vi "I2C.vi"() -> ()   [LabVIEW 2017]
doc: "Utilisez ce modèle pour construire un modèle de conception producteur/consommateur avec des événements et des files d'attente. Ce modèle est préférable à celui du Gestionnaire d'événements de l'interface utilisateur parce qu'il permet au code de s'exécuter de façon asynchrone en réponse à un événement, sans ralentir le temps de réponse de l'interface utilisateur."
uses:
  ctl/controle_boucle.ctl
panel:
  in  "adress":string
  in  "value (decimal":u8=255
  in  "hexa ?":bool
  in  "send":bool
  # "Adress"
  # "Data"
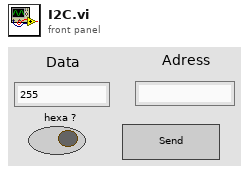
[diagram p1: front panel]
types:
  T1 = typedef "controle_boucle.ctl" = enum16{"stop", "Niveau 1", "Niveau 0"}
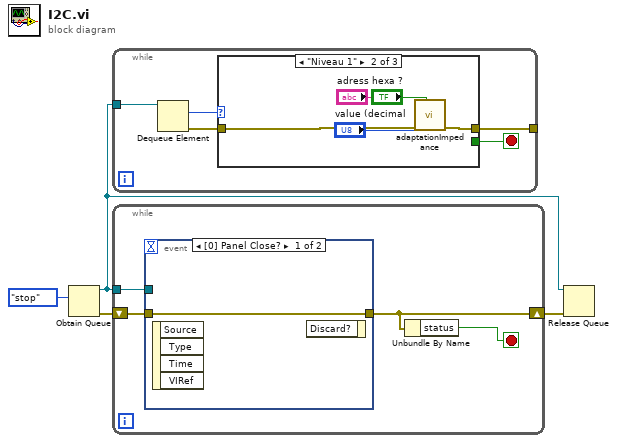
[diagram p0: block diagram]
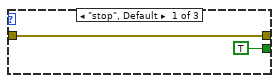
[diagram p2: hidden frame]
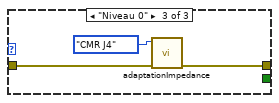
[diagram p3: hidden frame]
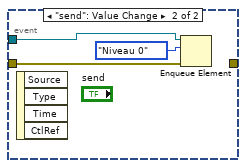
[diagram p4: hidden frame]
diagram:
  n1 = Obtain Queue(element data type=controle_boucle."stop") -> (queue out=w2:refnum<queue>, error out=w4:errorcluster)  [unwired: 4 in, 1 out]
  n2 = while {
    tunnel: w2 -> [w9]
    tunnel: [w5] -> _
    stop <- w8 stop-if-true
    n3 = Dequeue Element(queue=w9) -> (element=w7:T1, error out=w6:errorcluster)  [unwired: 2 in, 2 out]
    n4 = case shown="\"Niveau 1\"" w7 {
      tunnel: [TRUE _ _] -> w8
      tunnel: w6 -> [w10 w16 w18]
      tunnel: [w10 w15 w17] -> w5
      frame "stop", Default {
      }
      frame "Niveau 1" {
        n5 = call "adaptationImpedance.vi"("decimal / hexa"="hexa ?", "error in"=w16, "adress"="adress", "value (decimal"="value (decimal") -> ("error out"=w15:errorcluster)  [unwired: 7 in]
      }
      frame "Niveau 0" {
        n6 = call "adaptationImpedance.vi"("error in"=w18, "value (decimal"=enum16{"CMR J4", "Calibration coil"}."CMR J4" ("Énum")) -> ("error out"=w17:errorcluster)  [unwired: 9 in]
      }
    }
  }
  n7 = while {
    shift-right: [w21] -> w3
    shift-left: w4 -> [w22]
    tunnel: w2 -> [w23]
    stop <- w20 stop-if-true
    n8 = event shown="[0] Panel Close?" {
      selector: _ -> [_ _]
      dyn-events: _ -> [_ _]
      timeout: _ -> [_ _]
      tunnel: w23 -> [_ w26]
      tunnel: w22 -> [w24 w25]
      tunnel: [w24 _] -> w21
      event Panel Close? {
        n9 = event-data() -> ()  [unwired: 1 in, 4 out]
        n10 = event-data() -> ()  [unwired: 2 in, 1 out]
      }
      event "send": Value Change {
        n11 = event-data() -> ()  [unwired: 1 in, 4 out]
        n12 = Enqueue Element(queue=w26, element=controle_boucle."Niveau 0", error in (no error)=w25) -> ()  [unwired: 1 in, 3 out]
      }
    }
    n13 = Unbundle By Name(w21) -> ("status"=w20:bool)
  }
  n14 = Release Queue(queue=w2, error in (no error)=w3) -> ()  [unwired: 1 in, 3 out]
